vi "myoverlay_lines.vi"(4 "Color":u32(colorbox), 5 "Drawing Mode":u32(ring) items=["Frame", "Fill", "Highlight"], 8 "Line Endpoints":cluster{dbl, dbl}[](array[cluster]), 9 "Overlay Elements In":T1[](array[typedef]) {"Drawing Mode" items=["Frame", "Fill", "Highlight"]}) -> (3 "Overlay Elements Out":T1[](array[typedef]) {"Drawing Mode" items=["Frame", "Fill", "Highlight"]})   [LabVIEW 2010]
uses:
  overlay_element.ctl
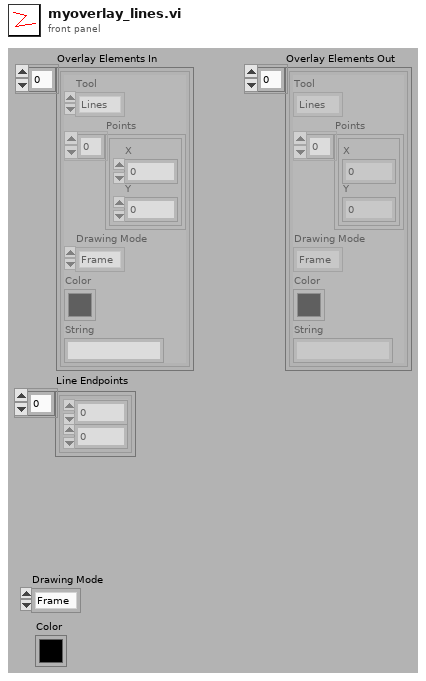
[diagram p1: front panel]
types:
  T1 = typedef "overlay_element.ctl" = cluster{"Tool":enum16{"Lines", "Oval", "Rectangle", "Text"}, "Points":cluster{"X":dbl, "Y":dbl}[], "Drawing Mode":u32, "Color":u32, "String":string}
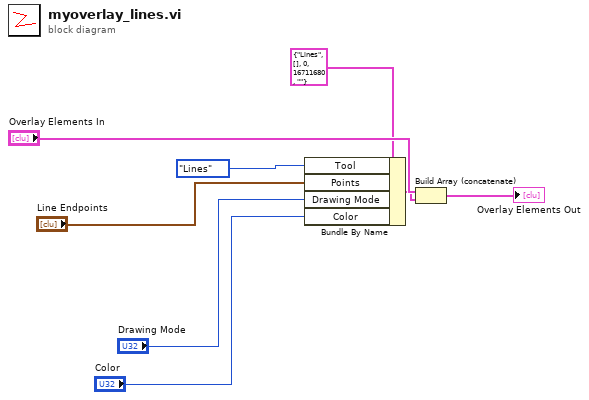
[diagram p0: block diagram]
diagram:
  n1 = Bundle By Name(cluster=T1 {"Tool"=enum."Lines", "Points"=[], "Drawing Mode"=0, "Color"=16711680, "String"=""} ("Cluster"), "Tool"=enum16{"Lines", "Oval", "Rectangle", "Text"}."Lines", "Points"="Line Endpoints", "Drawing Mode"="Drawing Mode", "Color"="Color") -> (w6:T1)
  n2 = Build Array (concatenate)("Overlay Elements In", w6) -> (→"Overlay Elements Out":T1[])
